vi "GetWaveforms.vi"(8 "error in (no error)":errorcluster, 11 "PmuTestFunctions in":refnum<class "ArbitraryFunction.lvclass">) -> (0 "error out":errorcluster, 2 "Waveforms":waveform(dbl)[](array[waveform]), 3 "PmuTestFunctions out":refnum<class "ArbitraryFunction.lvclass">)   [LabVIEW 2014, in "Functions.lvlib" / "ArbitraryFunction.lvclass"]
uses:
  ArbitraryFunction.lvclass
  ArbitraryFunction.lvclass/ArbitraryFunction.ctl
  Accessors/Read Arbs.vi
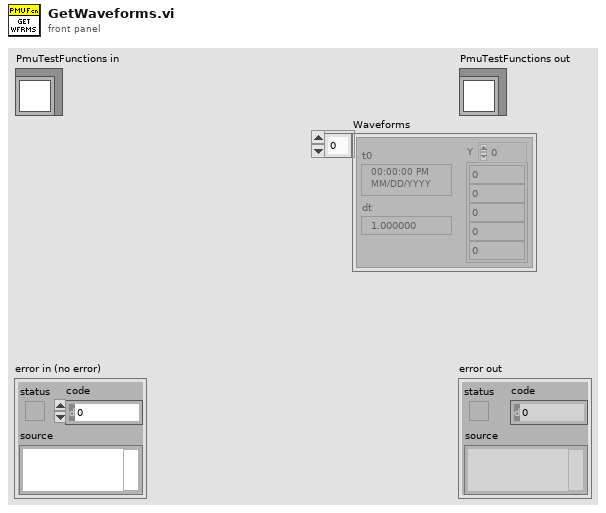
[diagram p1: front panel]
types:
  T1 = typedef "Functions.lvlib/ArbitraryFunction.lvclass/Arbitrary.ctl" = cluster{"Handle":string, "Size":i32, "Gain":dbl, "Offset":dbl, "Waveform":waveform(dbl)}
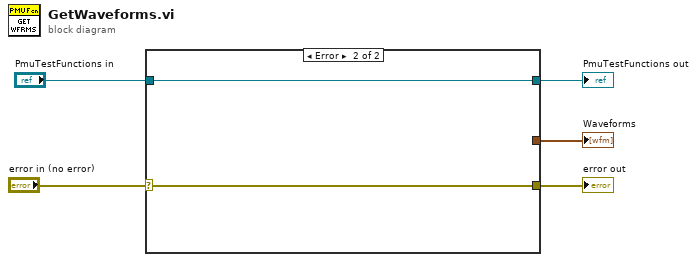
[diagram p0: block diagram]
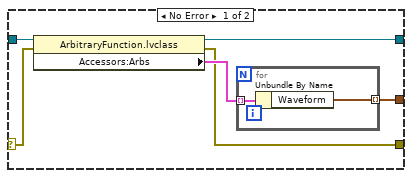
[diagram p2: hidden frame]
diagram:
  n1 = case shown="Error" "error in (no error)" {
    selector: "error in (no error)" -> [w8 w14]
    tunnel: [w6 w15] -> w3
    tunnel: "PmuTestFunctions in" -> [w11 w15]
    tunnel: [w7 w14] -> w2
    tunnel: [w9 _] -> w1
    frame No Error {
      n2 = property class="ArbitraryFunction.lvclass"(reference=w11, error in=w8) -> (reference out=w6:refnum<class "ArbitraryFunction.lvclass">, error out=w7:errorcluster, "Accessors:Arbs"=w10:T1[])
      n3 = for {
        tunnel: w10 -> [w13] mode=indexing
        tunnel: [w12] -> w9 mode=indexing
        n4 = Unbundle By Name(w13) -> ("Waveform"=w12:waveform(dbl))
      }
    }
    frame Error {
    }
  }
  "error out" <- w2
  "PmuTestFunctions out" <- w3
  "Waveforms" <- w1
